vi "specify execution settings.vi"(8 "error in":errorcluster, 10 "channels":refnum<class "TBM channel.lvclass">[](array[class]), 11 "fixed channel runtime in":refnum<class "CentralErrorHandler runtime.lvclass">) -> (0 "error out":errorcluster, 2 "execution settings":T1, 3 "fixed channel runtime out":refnum<class "CentralErrorHandler runtime.lvclass">)   [LabVIEW 2017, in "CentralErrorHandler runtime.lvclass"]
uses:
  CentralErrorHandler runtime.lvclass
  <vilib>/NI/Tag Bus Module Framework/runtime/execution settings.ctl
  <vilib>/NI/Tag Bus Module Framework/channel/TBM channel.lvclass
  <vilib>/NI/Tag Bus Module Framework/runtime/TBM module execution interface.lvclass
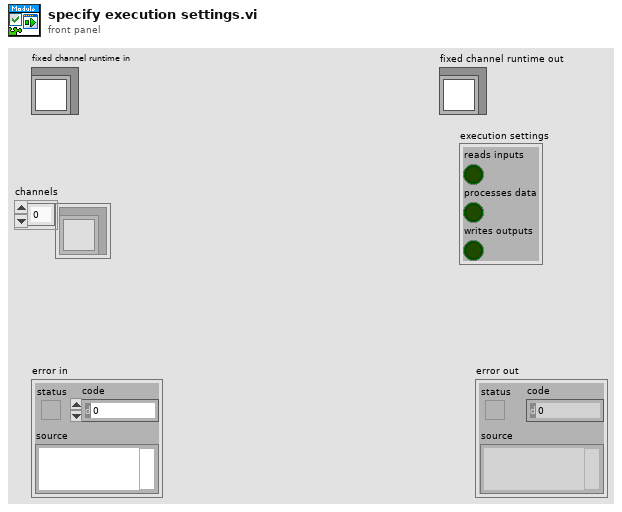
[diagram p1: front panel]
types:
  T1 = typedef "TBM module execution interface.lvclass/execution settings.ctl" = cluster{"reads inputs":bool, "processes data":bool, "writes outputs":bool}
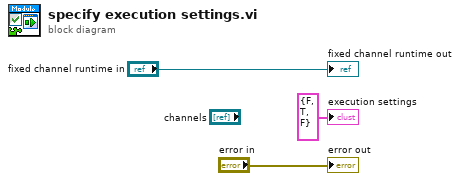
[diagram p0: block diagram]
diagram:
  "error out" <- "error in"
  "execution settings" <- T1 {"reads inputs"=FALSE, "processes data"=TRUE, "writes outputs"=FALSE} ("execution settings")
  "fixed channel runtime out" <- "fixed channel runtime in"
